vi "FSK_RFLoopback.vi"(5 "xsrpip":string, 7 "pcip":string, 8 "error in (no error)":errorcluster caption="错误输入（无错误）", 10 "SendSig":cdb[](array[numeric]), 11 "PathIn":path) -> (0 "error out":errorcluster caption="错误输出", 1 "ERR_CODE":dbl, 2 "RecvSig":cdb[](array[numeric]), 3 "PathOut":path)   [LabVIEW 2015]
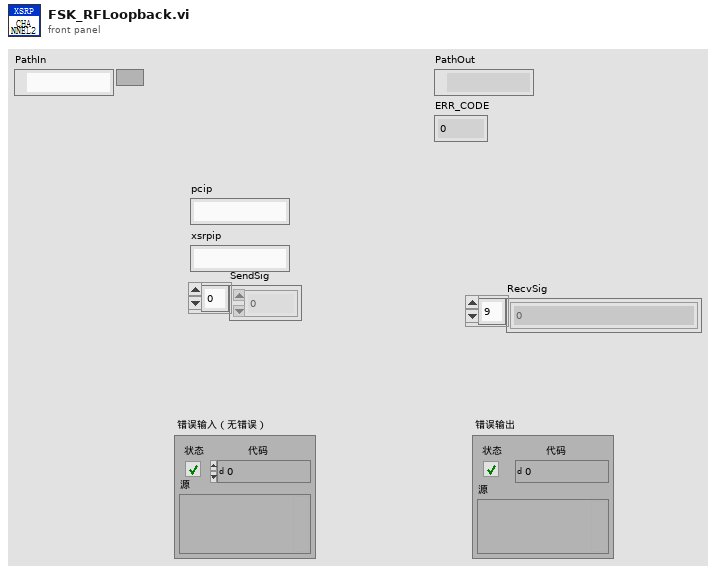
[diagram p1: front panel]
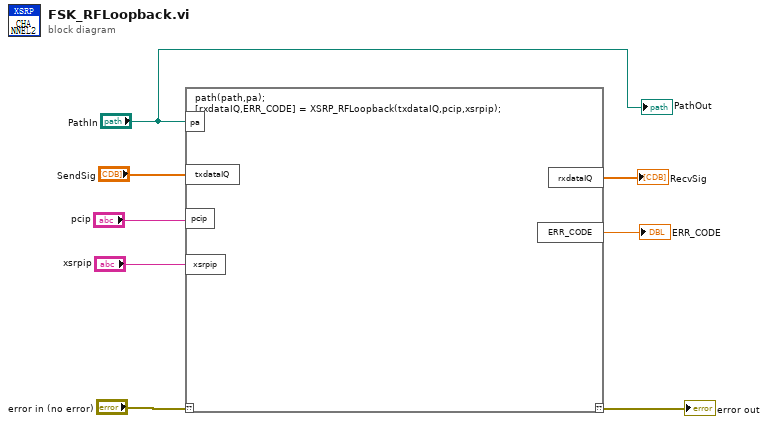
[diagram p0: block diagram]
diagram:
  n1 = script code="path(path,pa);\n[rxdataIQ,ERR_CODE] = XSRP_RFLoopback(txdataIQ,pcip,xsrpip);"("??"="error in (no error)", "pa"="PathIn", "txdataIQ"="SendSig", "xsrpip"="xsrpip", "pcip"="pcip") -> ("??"=→"error out":errorcluster, "rxdataIQ"=→"RecvSig":cdb[], "ERR_CODE"=→"ERR_CODE":dbl)
  "PathOut" <- "PathIn"
